vi "CurrentStep.vi"(8 "error in (no error)":errorcluster, 9 "index":i32, 11 "Array in":refnum<vi>) -> (0 "error out":errorcluster)   [LabVIEW 2019]
doc: "Mostra quale step sta venendo eseguito"
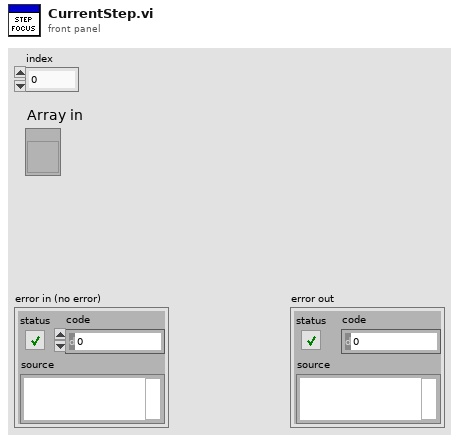
[diagram p1: front panel]
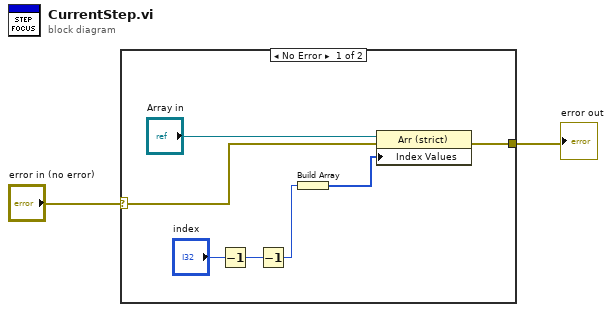
[diagram p0: block diagram]
diagram:
  n1 = case shown="No Error" "error in (no error)" {
    selector: "error in (no error)" -> [w9 w10]
    tunnel: [w8 w10] -> w1
    frame No Error {
      n2 = Decrement(x="index") -> (x-1=w5:i32)
      n3 = Decrement(x=w5) -> (x-1=w4:i32)
      n4 = Build Array(w4) -> (w7:i32[])
      n5 = property class="Arr (strict)"(reference="Array in", error in=w9, "Index Values"=w7) -> (error out=w8:errorcluster)  [unwired: 1 out]
    }
    frame Error {
    }
  }
  "error out" <- w1
